vi "Read_hardware.vi"(11 "configuration file path":path) -> (3 "data":T1)   [LabVIEW 2017]
uses:
  <vilib>/Utility/config.llb/NI_LVConfig.lvlib
panel:
  out "error out":errorcluster
  in  "error in (no error)":errorcluster
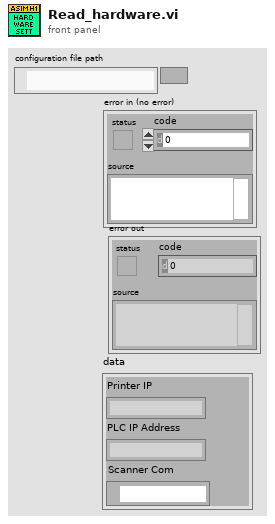
[diagram p1: front panel]
types:
  T1 = cluster{"Printer IP":string, "PLC IP Address":string, "Scanner Com":refnum<visa-resource-name>}
  T2 = typedef "NI_LVConfig.lvlib/Config Data RefNum.ctl" = refnum<k1>
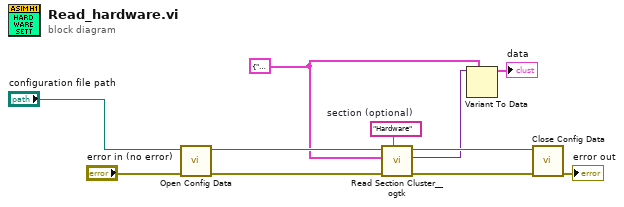
[diagram p0: block diagram]
diagram:
  w3 = T1 {"Printer IP"="", "PLC IP Address"="", "Scanner Com"=""}
  w9 = "Hardware"  # section (optional)
  n1 = call <vilib>:"Open Config Data.vi"("error in (no error)"="error in (no error)", "configuration file path"="configuration file path") -> ("error out"=w8:errorcluster, "refnum"=w11:T2)  [unwired: 7 in, 1 out]
  n2 = call <userlib>:"Read Section Cluster__ogtk.vi"("section (optional)"=w9, "error in (no error)"=w8, "Section Formatted Cluster Type"=w3, "refnum"=w11) -> ("error out"=w7:errorcluster, "Section Formatted Cluster"=w2:variant, "dup refnum"=w10:T2)  [unwired: 3 in, 2 out]
  n3 = Variant To Data(type=w3, Variant=w2) -> (data=→"data":T1)  [unwired: 1 in, 1 out]
  n4 = call <vilib>:"Close Config Data.vi"("error in (no error)"=w7, "refnum"=w10) -> ("error out"=→"error out":errorcluster)  [unwired: 8 in, 1 out]
